vi "AVQ8347 SRQ Signal Control 1.vi"(8 "Error In":errorcluster, 10 "SRQ Trans Sel (No Trans)":enum16{"No Trans", "Trans"}(ring), 11 "VISA Session":refnum<visa-resource-name>) -> (0 "Error Out":errorcluster, 2 "Send Code":string, 3 "Copy VISA Session":refnum<visa-resource-name>)   [LabVIEW 2020]
doc: "Selection of the transmission of SRQ"
panel:
  # "SRQ Signal Control 1"
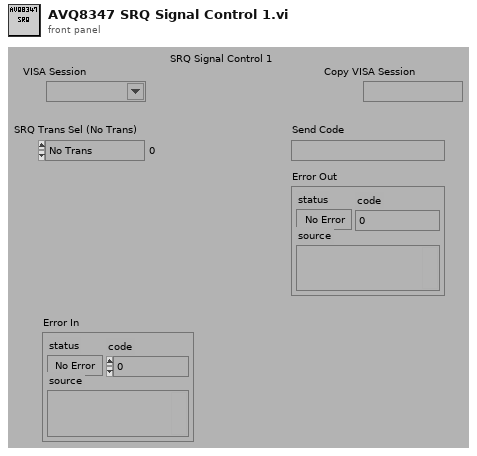
[diagram p1: front panel]
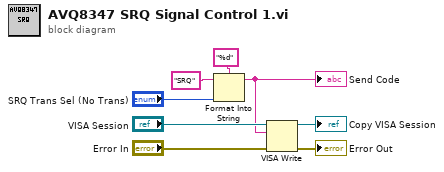
[diagram p0: block diagram]
diagram:
  n1 = Format Into String(format string="%d", initial string="SRQ", "SRQ Trans Sel (No Trans)") -> (resulting string=w1:string)  [unwired: 1 in, 1 out]
  "Send Code" <- w1
  n2 = VISA Write(VISA resource name="VISA Session", write buffer=w1, error in (no error)="Error In") -> (VISA resource name out=→"Copy VISA Session":refnum<visa-resource-name>, error out=→"Error Out":errorcluster)  [unwired: 1 out]
